vi "roboRIO v1.0 Unreserve AO.vi"(7 "Allow multiple opens?":bool, 8 "error in (no error)":errorcluster, 10 "AI Channel List":T1) -> (0 "error out":errorcluster)   [LabVIEW 2021]
uses:
  <vilib>/myRIO/Common/Instrument Driver Framework/myRIO v1.0/AO/typedefs/AO Channels List.ctl
  <vilib>/myRIO/Common/Instrument Driver Framework/myRIO v1.0/AO/typedefs/AO Channels Enum.ctl
  <vilib>/myRIO/Common/Instrument Driver Framework/roboRIO v1.0/Resource Manager/vis/roboRIO v1.0 Unreserve Channel.vi
  <vilib>/myRIO/Common/Instrument Driver Framework/roboRIO v1.0/Resource Manager/vis/roboRIO v1.0 Build Mutex Name.vi
  <vilib>/myRIO/Common/Instrument Driver Framework/Utilities/vis/Configuration Manager.vi
  <vilib>/myRIO/Common/Instrument Driver Framework/Utilities/vis/IO Manager.vi
  <vilib>/Utility/error.llb/Error Cluster From Error Code.vi
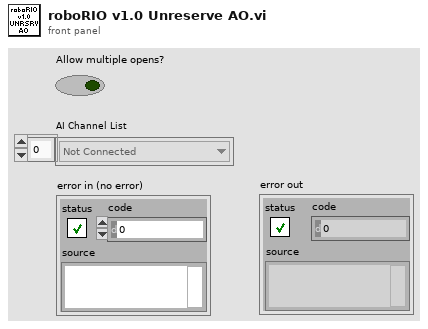
[diagram p1: front panel]
types:
  T1 = typedef "AO Channels List.ctl" = T2[]
  T2 = typedef "AO Channels Enum.ctl" = enum16{"Not Connected", "AudioOut/Left", "AudioOut/Right", "C/AO0", "C/AO1", "A/AO0", "A/AO1", "B/AO0", "B/AO1"}
  T3 = typedef "roboRIO v1.0 Channel Reservation List.ctl" = T4[]
  T4 = typedef "roboRIO v1.0 Channel Reservation Info.ctl" = cluster{"Channel Name":string, "Connector":T5, "Mutex ID":i32}
  T5 = typedef "roboRIO v1.0 Connector List.ctl" = enum32{"None", "ConnectorB", "ConnectorI2C", "ConnectorDIO", "ConnectorRSL", "ConnectorRELAY", "ConnectorAI", "ConnectorPWM", "ConnectorSPI"}
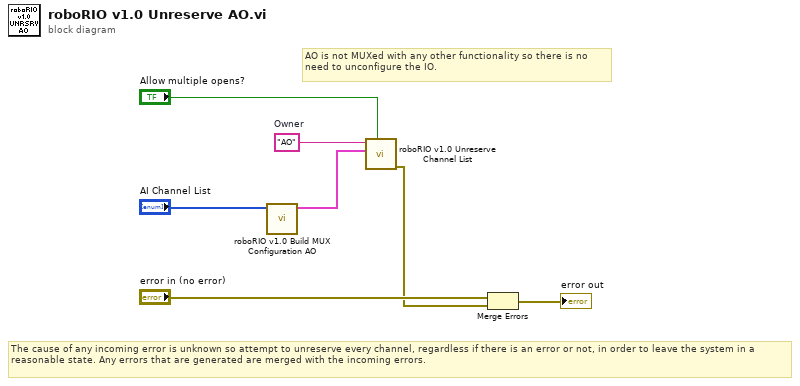
[diagram p0: block diagram]
diagram:
  w2 = "AO"  # Owner
  # "AO is not MUXed with any other functionality so there is no need to unconfigure the IO."
  # "The cause of any incoming error is unknown so attempt to unreserve every channel, regardless if there is an error or not, in order to leave the system in a reasonable state. Any errors that are generated are merged with the incoming errors."
  n1 = call <vilib>:"roboRIO v1.0 Build MUX Configuration AO.vi"("AO Channels List"="AI Channel List") -> ("Channel Reservation Info"=w3:T3)  [unwired: 10 in]
  n2 = call <vilib>:"roboRIO v1.0 Unreserve Channel List.vi"("Allow multiple opens?"="Allow multiple opens?", "Channel Reservation List"=w3, "Owner"=w2) -> ("error out"=w1:errorcluster)  [unwired: 8 in]
  n3 = Merge Errors("error in (no error)", w1) -> (→"error out":errorcluster)
